vi "SwitchAllianceColor.vi"(1 "Pressed":bool) -> ()   [LabVIEW 2020]
uses:
  <vilib>/Rock Robotics/Network Tables/NT Write Boolean.vi
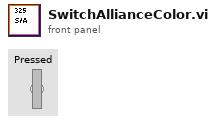
[diagram p1: front panel]
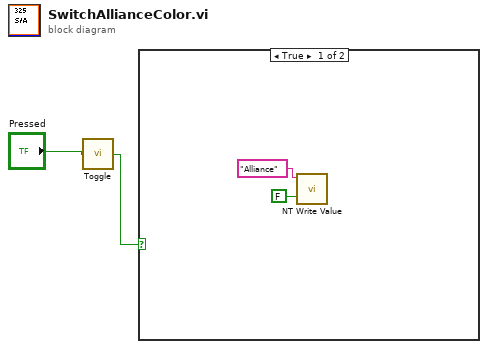
[diagram p0: block diagram]
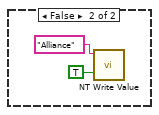
[diagram p2: hidden frame]
diagram:
  n1 = call "Toggle.vi"("Boolean"="Pressed") -> ("Boolean Out"=w1:bool)
  n2 = case shown="True" w1 {
    frame True {
      n3 = call-poly <vilib>:"NT Write Value.vi"("Boolean"=FALSE, "Name"="Alliance") -> ()  [unwired: 9 in, 1 out]
    }
    frame False {
      n4 = call-poly <vilib>:"NT Write Value.vi"("Boolean"=TRUE, "Name"="Alliance") -> ()  [unwired: 9 in, 1 out]
    }
  }
